vi "string_array_size_equal_to_zero.vi"(10 "array":string[](array[string])) -> (2 "size = 0?":bool)   [LabVIEW 2015]
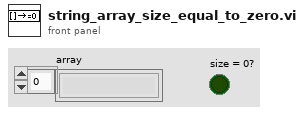
[diagram p1: front panel]
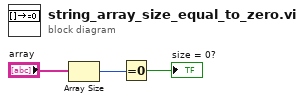
[diagram p0: block diagram]
diagram:
  n1 = Array Size(array="array") -> (size(s)=w2:i32)
  n2 = Equal To 0?(x=w2) -> (x = 0?=→"size = 0?":bool)
